vi "getImageNumber.vi"(8 "error in (no error)":errorcluster, 11 "WinX32Settings in":refnum<class "WinX32Settings.lvclass">) -> (0 "error out":errorcluster, 2 "image number":i32, 3 "WinX32Settings out":refnum<class "WinX32Settings.lvclass">)   [LabVIEW 2011, in "Tools.lvlib" / "Settings.lvlib" / "WinX32Settings.lvclass"]
uses:
  WinX32Settings.lvclass
  WinX32Settings.lvclass/WinX32Settings.ctl
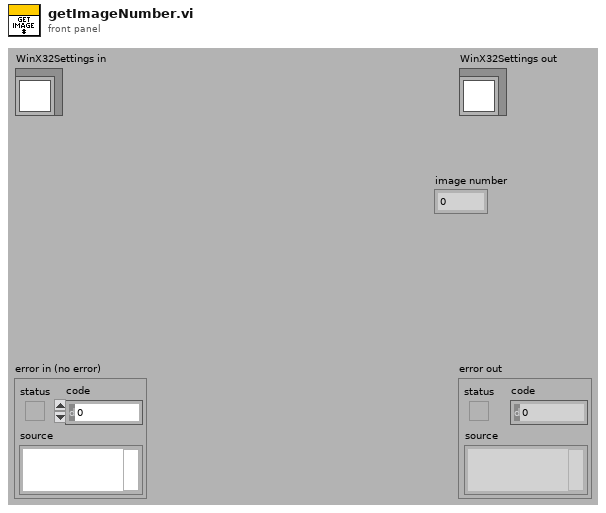
[diagram p1: front panel]
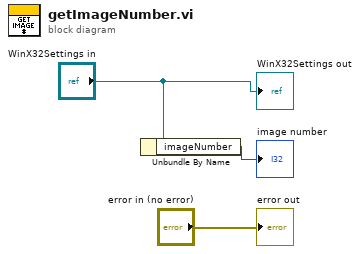
[diagram p0: block diagram]
diagram:
  n1 = Unbundle By Name("WinX32Settings in") -> ("imageNumber"=→"image number":i32)
  "error out" <- "error in (no error)"
  "WinX32Settings out" <- "WinX32Settings in"
